vi "NanotecSMCPDDriver.get reference status.vi"(0 "VISA resource name":refnum<visa-resource-name>, 1 "contollerID":i32=-1, 5 "error in (no error)":errorcluster) -> (14 "VISA resource name out":refnum<visa-resource-name>, 15 "contollerID out":i32=-1, 16 "referenced":u8, 19 "error out":errorcluster)   [LabVIEW 2015, in "NanotecSMCPDDriver.lvlib"]
doc: "Gets the reference status of the controller (1 = referenced)."
uses:
  NanotecSMCPDDriver.lvlib
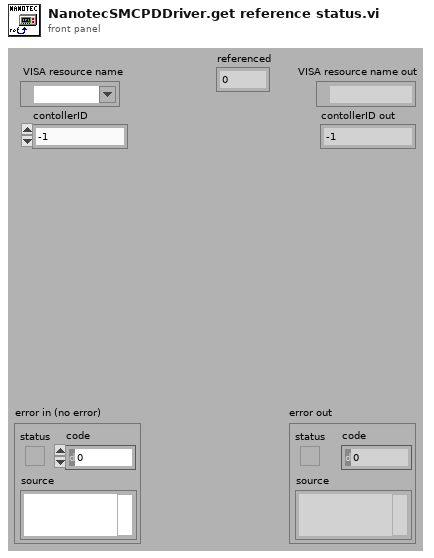
[diagram p1: front panel]
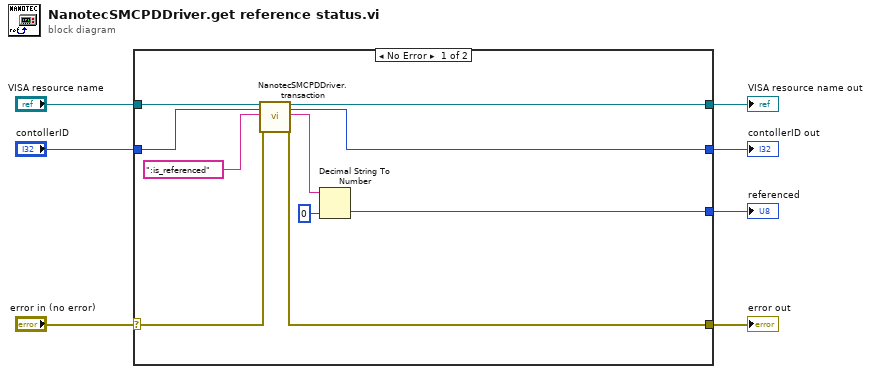
[diagram p0: block diagram]
diagram:
  n1 = case shown="No Error" "error in (no error)" {
    selector: "error in (no error)" -> [w10 w18]
    tunnel: [w13 w20] -> w7
    tunnel: [w11 w18] -> w6
    tunnel: "VISA resource name" -> [w17 w20]
    tunnel: "contollerID" -> [w15 w19]
    tunnel: [w14 w19] -> w3
    tunnel: [w9 _] -> w1
    frame No Error {
      n2 = call "NanotecSMCPDDriver.transaction.vi"("VISAresource"=w17, "contollerID"=w15, "commandString"=":is_referenced", "error in (no error)"=w10) -> ("VISAresource out"=w13:refnum<visa-resource-name>, "contollerID out"=w14:i32, "response"=w12:string, "error out"=w11:errorcluster)  [unwired: 10 in, 2 out]
      n3 = Decimal String To Number(string=w12, default (0L)=u8 0 ("default (0 I32)")) -> (number=w9:u8)  [unwired: 1 in, 1 out]
    }
    frame Error {
    }
  }
  "VISA resource name out" <- w7
  "error out" <- w6
  "contollerID out" <- w3
  "referenced" <- w1
